vi "SendCommandWithParameter.vi"(8 "Parameter":variant, 9 "Command":T1, 11 "Command Q":refnum<queue>) -> (3 "Command Q":refnum<queue>)   [LabVIEW 2013]
uses:
  Controls/ExperimentControlEnum.ctl
  Controls/ExperimentControlCluster.ctl
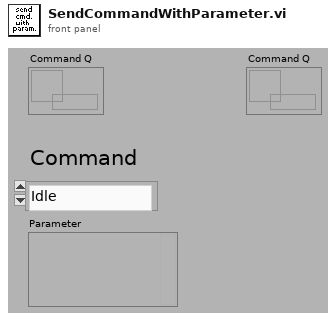
[diagram p1: front panel]
types:
  T1 = typedef "ExperimentControlEnum.ctl" = enum16{"Idle", "Software Start", "Load Init", "Bank Charging", "Trigger Start", "Trigger In Progress", "Acquire PXI Data", "Turn Off DIO", "Shot Log Save", "Clean Up", "Auto Updated", "Stop VI", "Adjust Bounds", "Update Shot", "Config Load", "Print VI", "Config Save As", "Timing Change", "Increment Timing", "DIO Change"}
  T2 = typedef "ExperimentControlCluster.ctl" = cluster{"Experiment Control":T1, "Variant":variant}
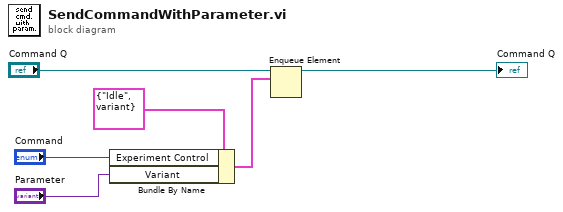
[diagram p0: block diagram]
diagram:
  n1 = Bundle By Name(cluster=T2 {"Experiment Control"=enum."Idle", "Variant"=variant} ("element"), "Experiment Control"="Command", "Variant"="Parameter") -> (w6:T2)
  n2 = Enqueue Element(queue="Command Q", element=w6) -> (queue out=→"Command Q":refnum<queue>)  [unwired: 1 in, 3 out]
